vi "ArmGlobal.vi"() -> ()   [LabVIEW 2023]
doc: "Arm global (getters and setter stuff)"
panel:
  out "ArmCalcSpeaker_Enabled":bool
  out "ArmPosition":dbl
  out "Arm2Position(Degrees)":dbl
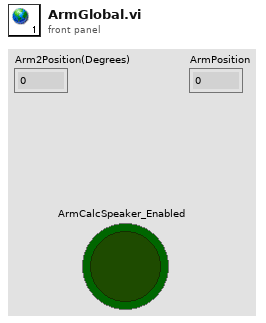
[diagram p1: front panel]
diagram:
